vi "Vacuum recording construct.vi"() -> ()   [LabVIEW 2015]
uses:
  <vilib>/platform/TimedLoop/XDataNode/XDataNode.xnode
  <vilib>/Platform/TimedLoop/XDataNode/nitl_modes.ctl
  <vilib>/Platform/TimedLoop/XDataNode/XDNodeRunTimeDep.lvlib
  <vilib>/Platform/TimedLoop/XDataNode/wakeup.ctl
  <vilib>/Platform/TimedLoop/XDataNode/timing_clust.ctl
panel:
  out "Waveform Graph":waveform(dbl)(graph)
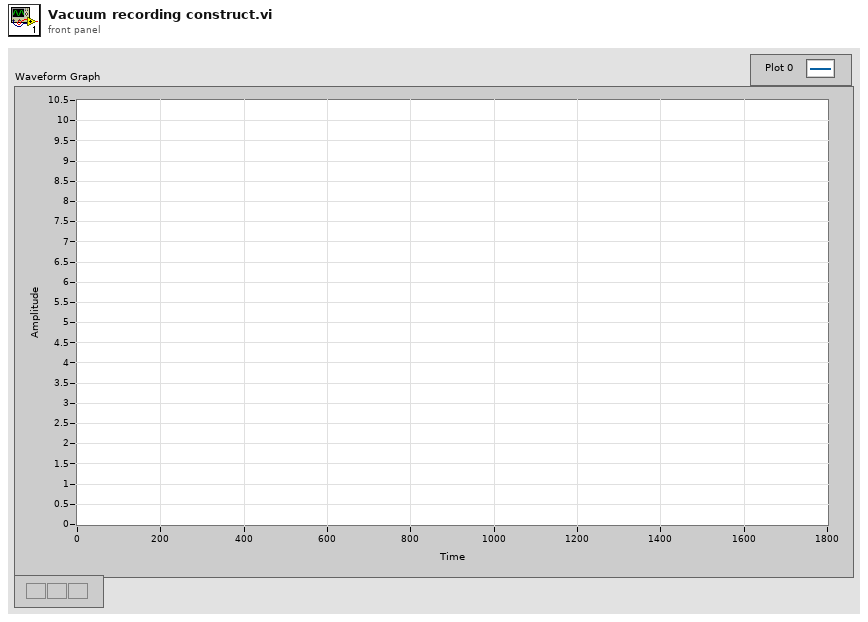
[diagram p1: front panel]
types:
  T1 = typedef "XDNodeRunTimeDep.lvlib/timing_clust.ctl" = cluster{"Expected End [f-1]":u64, "Actual End [f-1]":u64, "Finished Late? [f-1]":bool, "Expected End [i-1]":u64, "Actual End [i-1]":u64, "Finished Late? [i-1]":bool, "Expected Start [i]":u64, "Actual Start [i]":u64, "Expected Start [f]":u64, "Actual Start [f]":u64, "Source Name":string, "Structure Name":string, "Period":i64, "Deadline":i64, "Offset":i64, "Start":i64, "Priority":i32, "Timeout":i32, "Mode":T2, "Wakeup Reason":T3, "Error":errorcluster, "Source Type":string, "Secondary Source Type":string, "Global End Time":u64, "Global Start Time":u64, "Frame Duration":u64, "Iteration Duration":u64, "Assigned CPU":i32, "I/O Scan Engine Mode":u32}
  T2 = typedef "XDNodeRunTimeDep.lvlib/nitl_modes.ctl" = enum32{"No Change", "Process missed periods, maintain original phase", "Discard missed periods, maintain original phase", "Process missed periods, ignore original phase", "Discard missed periods, ignore original phase"}
  T3 = typedef "XDNodeRunTimeDep.lvlib/wakeup.ctl" = enum32{"Normal", "Aborted", "Asynchronous wakeup", "Timing source error", "Timed loop error", "Timeout"}
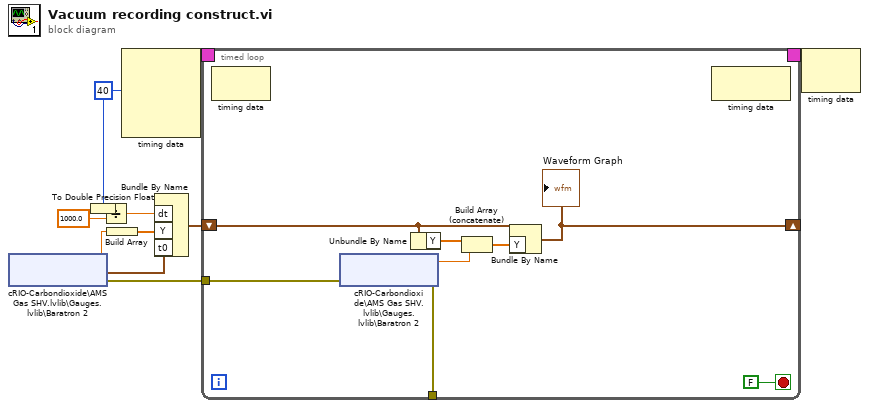
[diagram p0: block diagram]
diagram:
  w4 = i64 40 ("Period")
  n1 = shared-variable "cRIO-Carbondioxide\\AMS Gas SHV.lvlib\\Gauges.lvlib\\Baratron 2"() -> (w6:dbl, error out=w9:errorcluster, w7:timestamp)  [unwired: 1 in]
  n2 = To Double Precision Float(number=w4) -> (double precision float=w1:dbl)
  n3 = Divide(x=w1, y=1000.0) -> (x/y=w3:dbl)
  n4 = Build Array(w6) -> (w5:dbl[])
  n5 = node-c288(w4) -> (w11:T1)  [unwired: 3 in]
  n6 = Bundle By Name("dt"=w3, "Y"=w5, "t0"=w7) -> (w8:waveform(dbl))  [unwired: 1 in]
  n7 = timed-loop {
    timing: w11 -> [_]
    timing-out: [_] -> w10
    shift-right: [w12] -> _
    shift-left: w8 -> [w13]
    tunnel: [w18] -> _
    tunnel: w9 -> [w17]
    stop <- FALSE stop-if-true
    n8 = node-c288() -> ()  [unwired: 1 in, 1 out]
    n9 = shared-variable "cRIO-Carbondioxide\\AMS Gas SHV.lvlib\\Gauges.lvlib\\Baratron 2"(error in=w17) -> (w15:dbl, error out=w18:errorcluster)  [unwired: 1 out]
    n10 = Unbundle By Name(w13) -> ("Y"=w16:dbl[])
    n11 = Build Array (concatenate)(w16, w15) -> (w14:dbl[])
    n12 = Bundle By Name(cluster=w13, "Y"=w14) -> (w12:waveform(dbl))
    "Waveform Graph" <- w12
    n13 = node-c288() -> ()  [unwired: 1 in, 1 out]
  }
  n14 = node-c288(w10) -> ()  [unwired: 1 out]
